vi "PV ActiveLine - Language.vi"(7 "W/R":bool, 8 "Fehler (Eingang)":errorcluster, 9 "Language":u8(ring) items=["English (default)", "German", "French"], 11 "Referenz in":refnum<visa-resource-name>) -> (0 "Cluster (Ausgang)":errorcluster, 1 "Language ID":dbl, 2 "Language String":string, 3 "Referenz out":refnum<visa-resource-name>)   [LabVIEW 2013, in "PV ActiveLine.lvlib"]
doc: "LNG - Language\n\nReceive: a\n\nLanguage,\na =\n0 –> English (default)\n1 –> German\n2 –> French"
uses:
  <instrlib>/PV ActiveLine/PV ActiveLine.lvlib
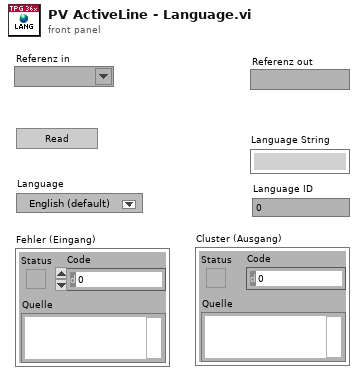
[diagram p1: front panel]
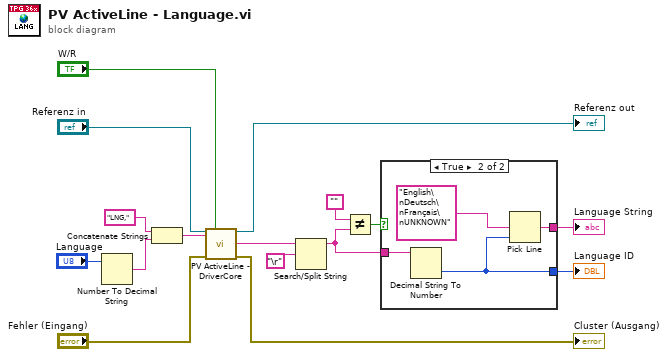
[diagram p0: block diagram]
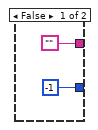
[diagram p2: hidden frame]
diagram:
  n1 = Number To Decimal String(number="Language") -> (decimal integer string=w10:string)  [unwired: 1 in]
  n2 = Concatenate Strings("LNG,", w10) -> (w12:string)
  n3 = call <instrlib>:"PV ActiveLine - DriverCore.vi"("Referenz in"="Referenz in", "Write/Read"="W/R", "Command"=w12, "Fehler (Eingang)"="Fehler (Eingang)") -> ("Referenz out"=→"Referenz out":refnum<visa-resource-name>, "String Out"=w14:string, "Cluster (Ausgang)"=→"Cluster (Ausgang)":errorcluster)  [unwired: 9 in]
  n4 = Search/Split String(string=w14, search string/char (-)="\r") -> (substring before match=w5:string)  [unwired: 1 in, 2 out]
  n5 = Not Equal?(x="", y=w5) -> (x != y?=w7:bool)
  n6 = case shown="True" w7 {
    tunnel: ["" w21] -> w6
    tunnel: w5 -> [_ w20]
    tunnel: [-1 w19] -> w4
    frame False {
    }
    frame True {
      n7 = Decimal String To Number(string=w20) -> (number=w19:i32)  [unwired: 2 in, 1 out]
      n8 = Pick Line(multi-line string="English\nDeutsch\nFrançais\nUNKNOWN", line index=w19) -> (output string=w21:string)  [unwired: 1 in]
    }
  }
  "Language String" <- w6
  "Language ID" <- w4
